vi "Set Phys Chan Property (1D I32).vi"(0 "session in":refnum<k21>, 5 "physical channels":refnum<k21>="$DefaultPhysChans", 7 "property":refnum<k21>, 9 "property value":i32[](array[numeric]), 11 "error in (no error)":errorcluster) -> (4 "session out":refnum<k21>, 15 "error out":errorcluster)   [LabVIEW 2020, in "SLSC.lvlib"]
doc: "Sets the value of the specified physical channel property for one or more physical channels to the provided value. Device-defined properties will not be written until a commit is called."
uses:
  <vilib>/SLSC/SLSC.lvlib
  nislsclvapi.dll
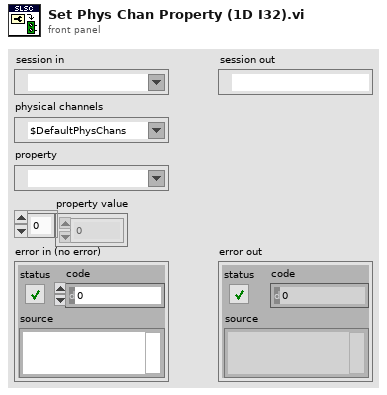
[diagram p1: front panel]
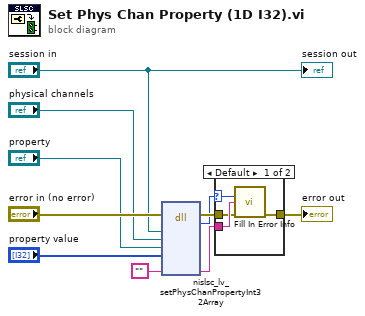
[diagram p0: block diagram]
diagram:
  n1 = dll-call lib="nislsclvapi.*" fn="nislsc_lv_setPhysChanPropertyInt32Array"(error in="error in (no error)", "session"="session in", "physChans"="physical channels", "property"="property", "propertyValue"="property value", "extendedErrorInfo"="") -> (error out=w7:errorcluster, w6:i32, "extendedErrorInfo"=w8:string)  [unwired: 8 in, 1 out]
  n2 = case shown="Default" w6 {
    selector: w6 -> [w14 _]
    tunnel: w8 -> [w13 _]
    tunnel: w7 -> [w12 w15]
    tunnel: [w11 w15] -> w5
    frame Default {
      n3 = call <vilib>:"Fill In Error Info.vi"("status code"=w14, "extended error info"=w13, "error in"=w12) -> ("error out"=w11:errorcluster)  [unwired: 12 in]
    }
    frame 0 {
    }
  }
  "error out" <- w5
  "session out" <- "session in"
